vi "Write_type.vi"(8 "error in (no error)":errorcluster, 10 "device type":string, 11 "PrepLinePictureObjects in":refnum<class "PrepLineObject.lvclass">) -> (0 "error out":errorcluster, 3 "PrepLinePictureObjects out":refnum<class "PrepLineObject.lvclass">)   [LabVIEW 2018, in "PrepLineObject.lvclass"]
doc: "sets the type of the PrepLine Picture Object (switch, pressure, temp)"
uses:
  PrepLineObject.lvclass
  PrepLineObject.lvclass/PrepLineObject.ctl
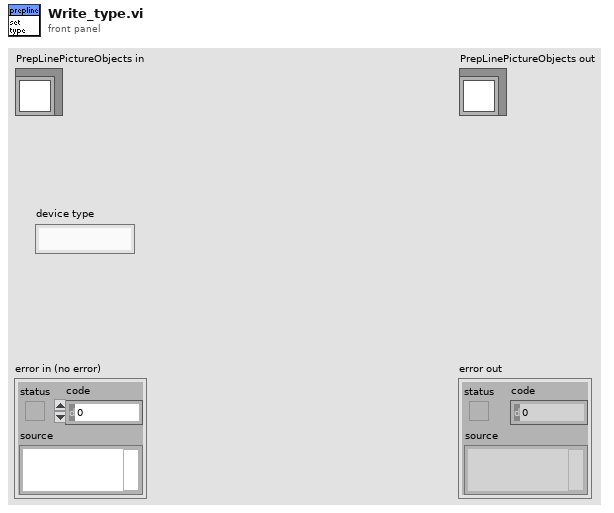
[diagram p1: front panel]
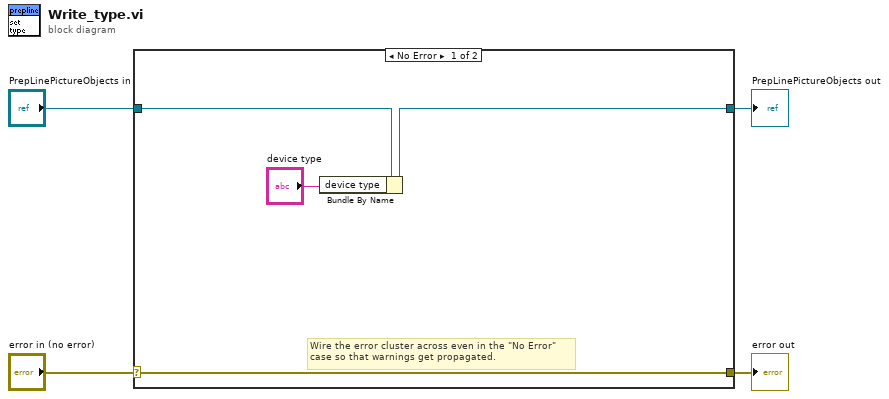
[diagram p0: block diagram]
diagram:
  n1 = case shown="No Error" "error in (no error)" {
    selector: "error in (no error)" -> [w7 w10]
    tunnel: [w7 w10] -> w3
    tunnel: [w6 w9] -> w1
    tunnel: "PrepLinePictureObjects in" -> [w8 w9]
    frame No Error {
      # "Wire the error cluster across even in the \"No Error\"\ncase so that warnings get propagated."
      n2 = Bundle By Name(cluster=w8, "device type"="device type") -> (w6:refnum<class "PrepLineObject.lvclass">)
    }
    frame Error {
    }
  }
  "error out" <- w3
  "PrepLinePictureObjects out" <- w1
